vi "interpolate and convert for graph.vi"(10 "Array":dbl[](array[numeric]), 11 "a_pWaveLength":dbl[](array[numeric])) -> (3 "XY Graph":cluster{"X":dbl, "Y":dbl}[](graph))   [LabVIEW 2013]
uses:
  <vilib>/Analysis/1siggen.llb/Ramp Pattern by Delta.vi
  <vilib>/gmath/NI_Gmath.lvlib
  <vilib>/Analysis/NI_AALBase.lvlib
panel:
  out "size(s) 2":i32
  out "size(s)":i32
  out "error":i32
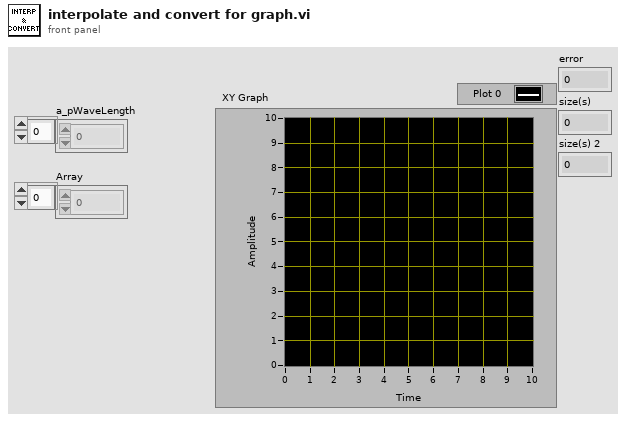
[diagram p1: front panel]
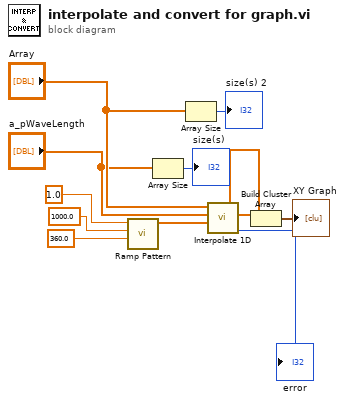
[diagram p0: block diagram]
diagram:
  n1 = call-poly <vilib>:"Ramp Pattern.vi"("start"=360.0, "end"=1000.0, "delta"=1.0) -> ("Ramp Pattern"=w12:dbl[])  [unwired: 6 in, 2 out]
  n2 = Array Size(array="a_pWaveLength") -> (size(s)=→"size(s)":i32)
  n3 = Array Size(array="Array") -> (size(s)=→"size(s) 2":i32)
  n4 = call <vilib>:"Interpolate 1D.vi"("xi"=w12, "X"="a_pWaveLength", "Y"="Array") -> ("error"=→"error":i32, "xi used"=w8:dbl[], "yi"=w7:dbl[])  [unwired: 6 in]
  n5 = Build Cluster Array(w8, w7) -> (→"XY Graph":cluster{"Numeric":dbl, "Numeric":dbl}[])
